vi "Start Laser.vi"(8 "error in (no error)":errorcluster, 11 "Test Station SIM Laser Driver in":refnum<class "Test Station SIM Laser Driver.lvclass">) -> (0 "error out":errorcluster, 3 "Test Station SIM Laser Driver out":refnum<class "Test Station SIM Laser Driver.lvclass">)   [LabVIEW 2022 SP3, in "Test Station SIM Laser Driver.lvclass"]
uses:
  Test Station SIM Laser Driver.lvclass
  Sim Laser Driver/Sim Laser Driver.lvclass
  Test Station SIM Laser Driver.lvclass/Test Station SIM Laser Driver.ctl
  Action.ctl
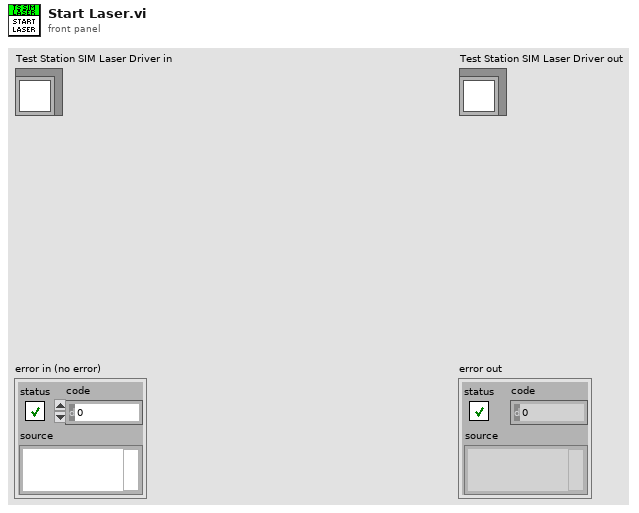
[diagram p1: front panel]
types:
  T1 = typedef "Test Station SIM Laser Driver.lvclass/Action.ctl" = enum16{"Read Data", "Set Data"}
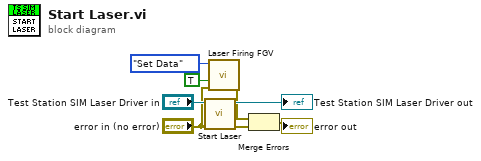
[diagram p0: block diagram]
diagram:
  n1 = call-parent "Start Laser.vi"("error in (no error)"="error in (no error)", "Sim Laser Driver in"="Test Station SIM Laser Driver in") -> ("error out"=w8:errorcluster, "Sim Laser Driver out"=→"Test Station SIM Laser Driver out":refnum<class "Test Station SIM Laser Driver.lvclass">)  [unwired: 8 in]
  n2 = call "Laser Firing FGV.vi"("error in (no error)"="error in (no error)", "Laser Firing"=TRUE, "Action"=Action."Set Data") -> ("error out"=w1:errorcluster)  [unwired: 7 in, 1 out]
  n3 = Merge Errors(w1, w8) -> (→"error out":errorcluster)
